vi "VI Server_OpenDecorationRefs.vi"(6 "Decoration Labels":string[](array[string]), 7 "Tab.Labels":string[](array[string]), 8 "error in":errorcluster, 11 "VI Server Cluster":T1) -> (0 "error out":errorcluster, 3 "VI Server Cluster.DUP":T1 caption="VI Server Cluster.OUT", 4 "Decorations.Cluster":T2)   [LabVIEW 2020]
uses:
  VI Server_TypeDefs/VI Server_Decorations_Cluster.ctl
  VI Server_TypeDefs/VI Server_RefsCluster.ctl
  toolkits_lv2020_32bit/Synchronization.llb/SynchRefs_SetGet.ctl
  VI Server Toolkit LV2013.lvlib
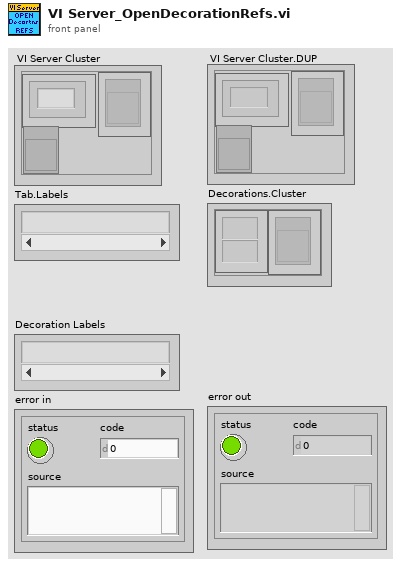
[diagram p1: front panel]
types:
  T1 = typedef "VI Server_RefsCluster.ctl" = cluster{"Labels":string[], "Refs":refnum<vi>[], "VI Ref":refnum<vi>}
  T2 = typedef "VI Server_Decorations_Cluster.ctl" = cluster{"Decoration Labels":string[], "Decorations[].Refs":refnum<vi>[]}
  T3 = typedef "SynchRefs_SetGet.ctl" = enum16{"Set", "Get"}
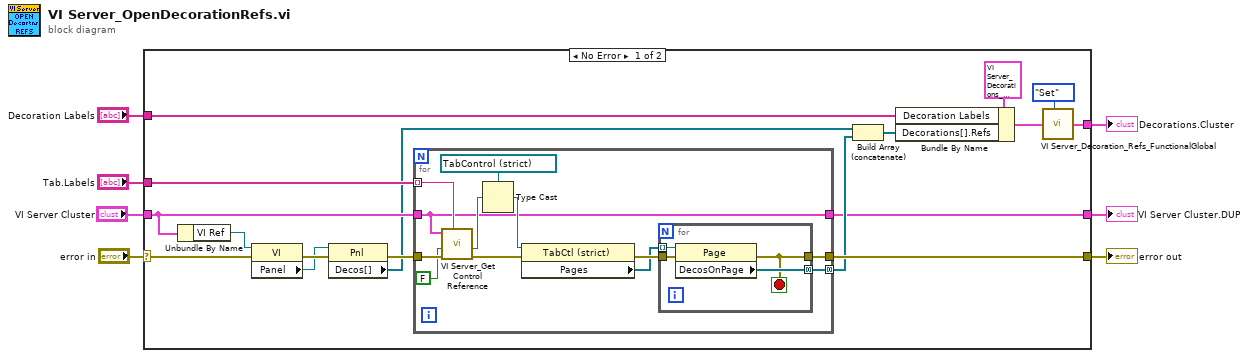
[diagram p0: block diagram]
diagram:
  n1 = case shown="No Error" "error in" {
    selector: "error in" -> [w17 w41]
    tunnel: [w14 w41] -> w6
    tunnel: "Decoration Labels" -> [w21 _]
    tunnel: [w18 _] -> w4
    tunnel: "VI Server Cluster" -> [w13 _]
    tunnel: "Tab.Labels" -> [w12 _]
    tunnel: [w8 _] -> w1
    frame No Error {
      n2 = Unbundle By Name(w13) -> ("VI Ref"=w16:refnum<vi>)
      n3 = property class="VI"(reference=w16, error in=w17) -> (error out=w24:errorcluster, "Panel"=w23:refnum<vi>)  [unwired: 1 out]
      n4 = property class="Pnl"(reference=w23, error in=w24) -> (error out=w15:errorcluster, "Decos[]"=w11:refnum<vi>[])  [unwired: 1 out]
      n5 = for {
        tunnel: w13 -> [w26]
        tunnel: w12 -> [w31] mode=indexing
        tunnel: w15 -> [w32]
        tunnel: [w28] -> w14
        tunnel: [w27] -> w10 mode=concatenating
        tunnel: [w26] -> w8
        n6 = call "VI Server_Get Control Reference.vi"("Label"=w31, "error in"=w32, "Single Instance (T)"=FALSE, "VI Server Cluster"=w26) -> ("error out"=w34:errorcluster, "Control Reference (Generic)"=w36:refnum<vi>)  [unwired: 6 out]
        n7 = Type Cast(type=refnum<vi> refnum ("TabCtlRef"), x=w36) -> (*(type *) &x=w35:refnum<vi>)
        n8 = property class="TabCtl (strict)"(reference=w35, error in=w34) -> (error out=w30:errorcluster, "Pages"=w29:refnum<vi>[])  [unwired: 1 out]
        n9 = for {
          tunnel: w30 -> [w40]
          tunnel: w29 -> [w39] mode=indexing
          tunnel: [w38] -> w27 mode=concatenating
          tunnel: [w37] -> w28
          stop <- w37 stop-if-true
          n10 = property class="Page"(reference=w39, error in=w40) -> (error out=w37:errorcluster, "DecosOnPage"=w38:refnum<vi>[])  [unwired: 1 out]
        }
      }
      n11 = Build Array (concatenate)(w11, w10) -> (w9:refnum<vi>[])
      n12 = Bundle By Name(cluster=T2 {"Decoration Labels"=[], "Decorations[].Refs"=[refnum, refnum, refnum, refnum, refnum, refnum, refnum, refnum, refnum, refnum]} ("Decorations.Cluster"), "Decoration Labels"=w21, "Decorations[].Refs"=w9) -> (w19:T2)
      n13 = call "VI Server_Decoration_Refs_FunctionalGlobal.vi"("SynchRefs.Set/Get"=SynchRefs_SetGet."Set", "SynchRefs.IN"=w19) -> ("SynchRefs.OUT"=w18:T2)  [unwired: 5 in]
    }
    frame Error {
    }
  }
  "error out" <- w6
  "Decorations.Cluster" <- w4
  "VI Server Cluster.DUP" <- w1
